vi "alg_special (SubVI).vi"(8 "에러 입력(에러 없음)":errorcluster, 10 "matrix size":i32, 11 "matrix type":i32(ring)=1 items=["zeros", "단위"]) -> (0 "에러 출력":errorcluster, 2 "ans":dbl[][](array[numeric])=[[1.0, 2.0], [3.0, 4.0]], 3 "참조 번호 출력":refnum<k35>)   [LabVIEW 2018]
uses:
  PythonConfigGlobal.vi
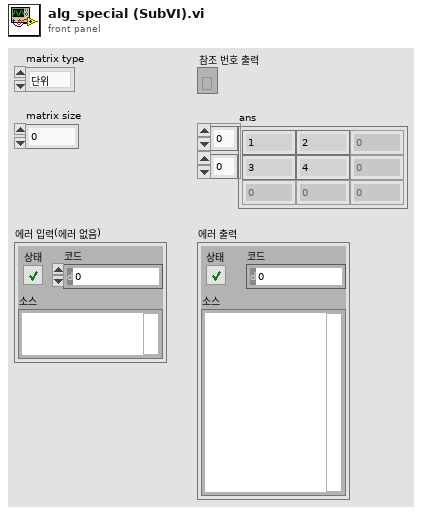
[diagram p1: front panel]
types:
  T1 = cluster{"session out":refnum<k35>, "appended path":path}
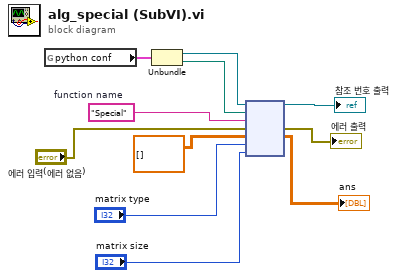
[diagram p0: block diagram]
diagram:
  w4 = "Special"  # function name
  n1 = global read "PythonConfigGlobal.vi" "python conf"() -> (w7:T1)
  n2 = Unbundle(w7) -> ("session out"=w5:refnum<k35>, "appended path"=w6:path)
  n3 = node(w5, w6, w4, "에러 입력(에러 없음)", dbl[][] [] ("str1"), "matrix type", "matrix size") -> (→"참조 번호 출력":refnum<k35>, →"에러 출력":errorcluster, →"ans":dbl[][])  [unwired: 2 in, 2 out]
